vi "编辑选中文件.vi"() -> ()   [LabVIEW 2015]
panel:
  in  "文件类型":string="*.txt"
  in  "路径":path=path "F:/LabVIEW 2014中文版  尚晨/yuanwenjian/8/8.2"
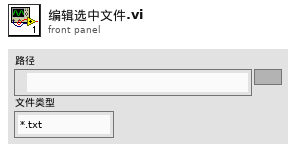
[diagram p1: front panel]
types:
  T1 = enum16{"Left Button", "Center Button", "Right Button", "Window Close"}
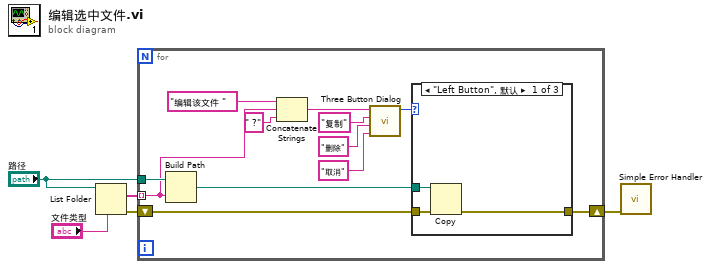
[diagram p0: block diagram]
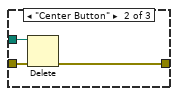
[diagram p2: hidden frame]
diagram:
  n1 = List Folder ("List Directory")(path="路径", pattern="文件类型") -> (filenames=w4:string[], error out=w2:errorcluster)  [unwired: 1 in, 3 out]
  n2 = for {
    tunnel: w4 -> [w11] mode=indexing
    tunnel: "路径" -> [w12]
    shift-right: [w9] -> w1
    shift-left: w2 -> [w8]
    n3 = Build Path(base path=w12, name or relative path=w11) -> (appended path=w10:path)
    n4 = Concatenate Strings("编辑该文件 " ("Substring"), w11, " ?" ("Substring")) -> (w14:string)
    n5 = call <vilib>:"Three Button Dialog.vi"("Right Button Text (\"Cancel\")"="取消" ("F button name (\"Cancel\")"), "Center Button Text (\"No\")"="删除" ("T button name (\"OK\")"), "Left Button Text (\"Yes\")"="复制" ("Left Button Text (\"Yes\")"), "message"=w14) -> ("Which Button?"=w15:T1)  [unwired: 7 in]
    n6 = case shown="\"Left Button\", 默认" w15 {
      tunnel: w10 -> [w18 w23 _]
      tunnel: [w19 w22 w24] -> w9
      tunnel: w8 -> [w20 w21 w24]
      frame "Left Button", Default {
        n7 = Copy(8:w20, 11:w18) -> (0:w19:errorcluster)  [unwired: 3 in, 2 out]
      }
      frame "Center Button" {
        n8 = Delete(path (use dialog)=w23, error in=w21) -> (error out=w22:errorcluster)  [unwired: 5 out]
      }
      frame "Right Button" {
      }
    }
  }
  n9 = call <vilib>:"Simple Error Handler.vi"("error in (no error)"=w1) -> ()  [unwired: 1 in, 8 out]
